vi "resetOutput.vi"(8 "error in (no error)":errorcluster, 11 "HamegHMPSupply in":refnum<class "HamegHMPSupply.lvclass">) -> (0 "error out":errorcluster, 3 "HamegHMPSupply out":refnum<class "HamegHMPSupply.lvclass">)   [LabVIEW 2011, in "Hardware.lvlib" / "Channels.lvlib" / "HamegHMPSupply.lvclass"]
uses:
  HamegHMPSupply.lvclass
  AnalogOutput.lvclass
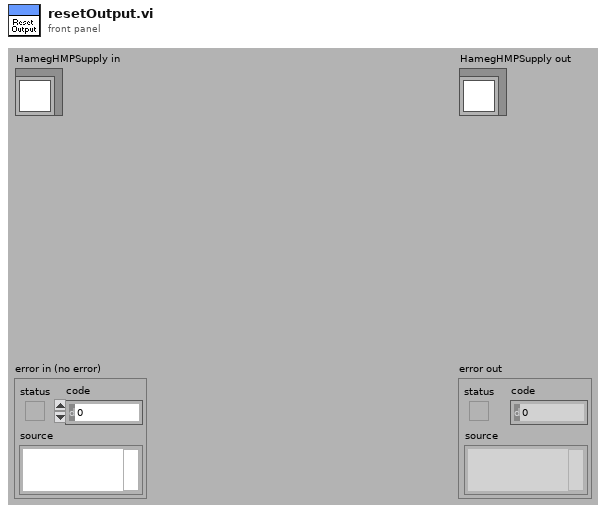
[diagram p1: front panel]
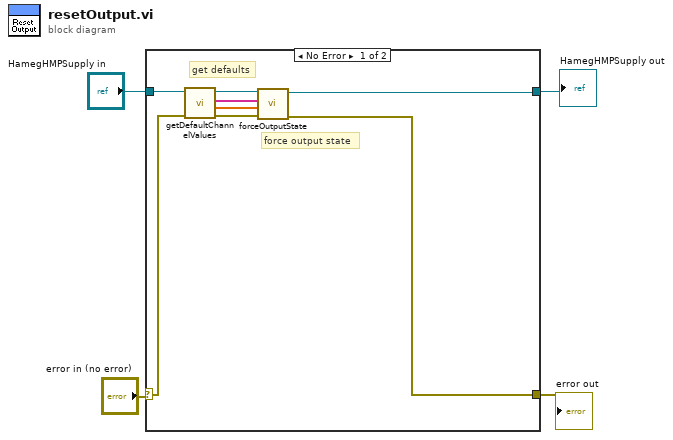
[diagram p0: block diagram]
diagram:
  n1 = case shown="No Error" "error in (no error)" {
    selector: "error in (no error)" -> [w11 w14]
    tunnel: "HamegHMPSupply in" -> [w12 w13]
    tunnel: [w5 w14] -> w2
    tunnel: [w6 w13] -> w1
    frame No Error {
      # "get defaults"
      # "force output state"
      n2 = call "getDefaultChannelValues.vi"("error in (no error)"=w11, "AnalogOutput in"=w12) -> ("error out"=w7:errorcluster, "calibratedValues"=w8:dbl[], "channel_addresses"=w9:string[], "AnalogOutput out"=w10:refnum<class "HamegHMPSupply.lvclass">)  [unwired: 6 in]
      n3 = call-dynamic "forceOutputState.vi"("error in (no error)"=w7, "calibratedValues"=w8, "channel_addresses"=w9, "HamegHMPSupply in"=w10) -> ("error out"=w5:errorcluster, "HamegHMPSupply out"=w6:refnum<class "HamegHMPSupply.lvclass">)  [unwired: 6 in]
    }
    frame Error {
    }
  }
  "error out" <- w2
  "HamegHMPSupply out" <- w1
